vi "CliffLogic.vi"(10 "State In":string, 11 "Light Threshold":sgl) -> (0 "Both Light":bool, 1 "Right Light":bool, 2 "Left Light":bool, 3 "State Out":string)   [LabVIEW 2016, in "SumoRobot.lvrbt"]
uses:
  SumoRobot.lvrbt
  <vilib>/NXT/Block Support/NXT_InputPort.ctl
  <vilib>/NXT/Dual Mode Library/Sensors/EV3_Color_Reflect.vi
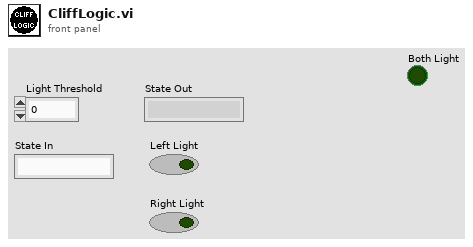
[diagram p1: front panel]
types:
  T1 = typedef "NXT_InputPort.ctl" = u32
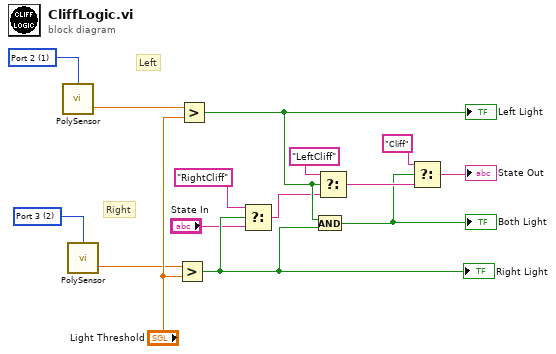
[diagram p0: block diagram]
diagram:
  w8 = T1 2 items=["Port 1", "Port 2", "Port 3", "Port 4"] ("Port (Port 1)")
  w5 = T1 1 items=["Port 1", "Port 2", "Port 3", "Port 4"] ("Port (Port 1)")
  # "Right"
  # "Left"
  n1 = call-poly <vilib>:"PolySensor.vi"("Port (Port 1)"=w5) -> ("Scaled Value"=w6:sgl)  [unwired: 2 in, 1 out]
  n2 = call-poly <vilib>:"PolySensor.vi"("Port (Port 1)"=w8) -> ("Scaled Value"=w7:sgl)  [unwired: 2 in, 1 out]
  n3 = Greater?(x=w7, y="Light Threshold") -> (0:w4:bool)
  "Right Light" <- w4
  n4 = Greater?(x=w6, y="Light Threshold") -> (0:w11:bool)
  "Left Light" <- w11
  n5 = Select(t="RightCliff", s=w4, f="State In") -> (s? t:f=w3:string)
  n6 = And(x=w11, y=w4) -> (x .and. y?=w12:bool)
  "Both Light" <- w12
  n7 = Select(t="LeftCliff", s=w11, f=w3) -> (s? t:f=w13:string)
  n8 = Select(t="Cliff", s=w12, f=w13) -> (s? t:f=→"State Out":string)
